vi "1_OnInterrupts.vi"() -> ()   [LabVIEW 2020]
uses:
  <vilib>/Instr/_visa.llb/VISA Configure Serial Port (Instr).vi
  <vilib>/Analysis/NI_AALBase.lvlib
panel:
  in  "stop":bool
  in  "Tab Control":enum32{"Main", "Service"}(tab)
  out "mean":dbl=672.206 format="%.6f"
  out "standard deviation":dbl=7.149110683653894 format="%.6f"
  out "Measurement":dbl(graph)=673.0
  out "error out":errorcluster
  in  "VISA resource name":refnum<visa-resource-name>="COM7"
  out "answer":string="673 \n\r"
  in  "Clear":bool
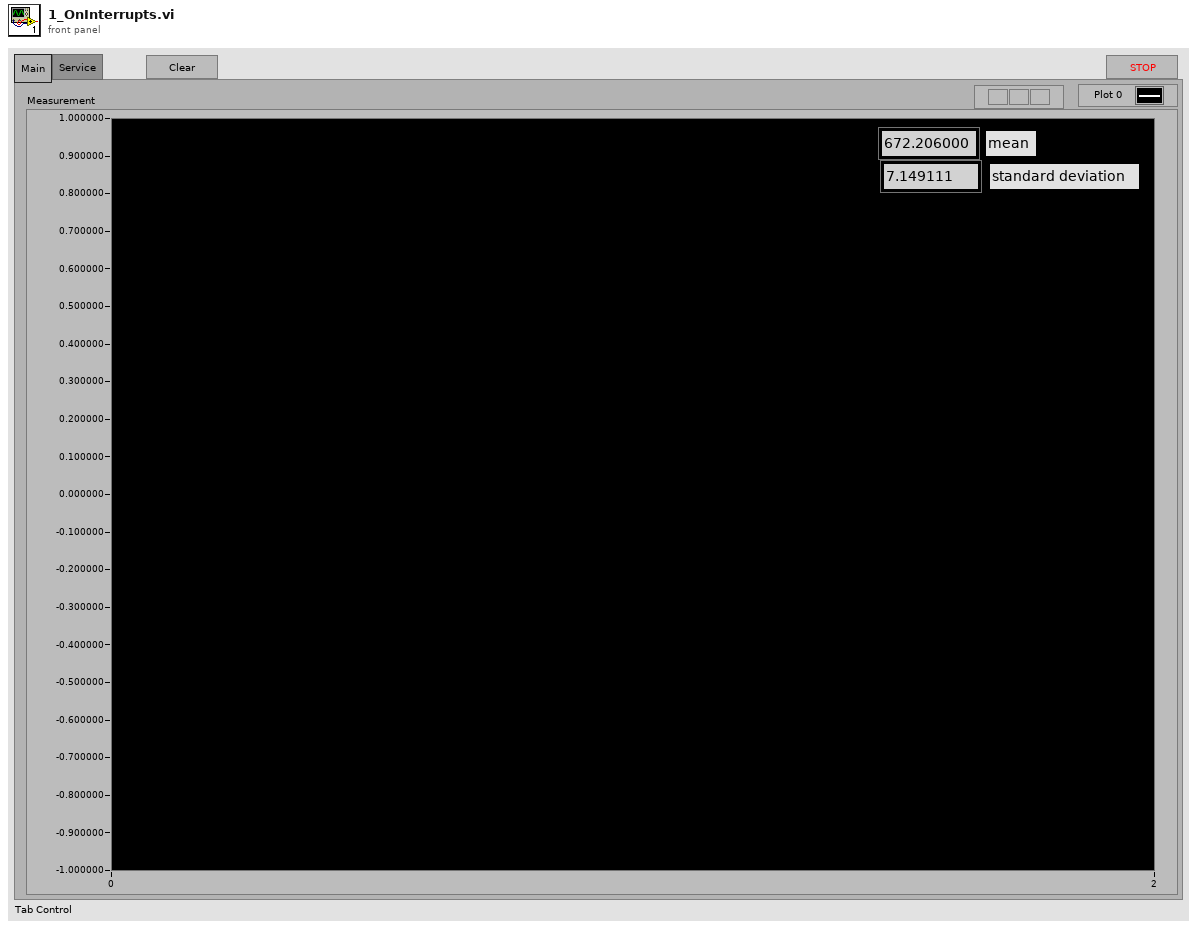
[diagram p1: front panel]
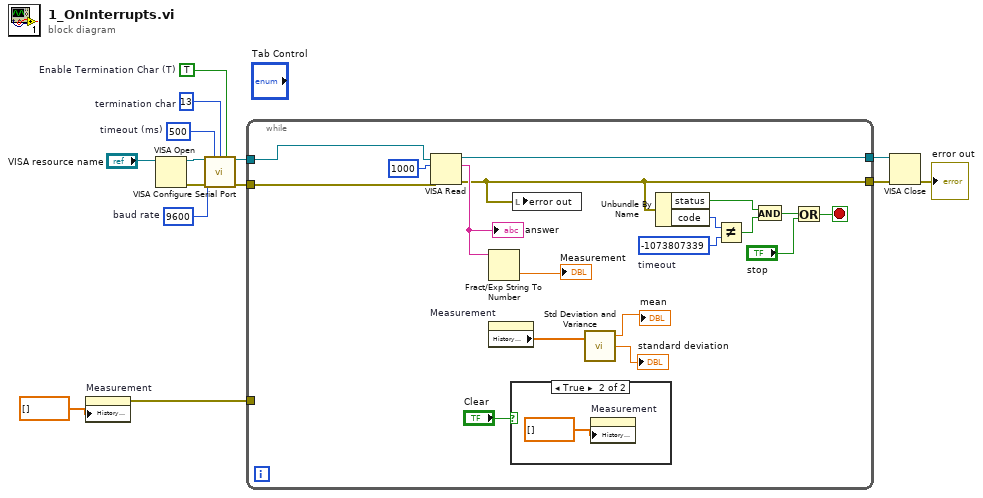
[diagram p0: block diagram]
diagram:
  w3 = u32 9600  # baud rate
  w4 = u32 500  # timeout (ms)
  w10 = TRUE  # Enable Termination Char (T)
  w11 = u8 13  # termination char
  n1 = property on="Measurement" class="WFChart (strict)"("History Data"=dbl[] []) -> (error out=w1:errorcluster)  [unwired: 2 in, 1 out]
  n2 = VISA Open(VISA resource name="VISA resource name") -> (VISA resource name=w13:refnum<visa-resource-name>, error out=w14:errorcluster)  [unwired: 4 in]
  n3 = call-poly "VISA Configure Serial Port"("VISA resource name"=w13, "timeout (10sec)"=w4, "termination char\n(0xA = '\\n' = LF)"=w11, "Enable Termination\nChar (T)"=w10, "baud rate (9600)"=w3, "error in (no error)"=w14) -> ("VISA resource name out"=w7:refnum<visa-resource-name>, "error out"=w6:errorcluster)  [unwired: 8 in]
  n4 = while {
    tunnel: w7 -> [w31]
    tunnel: [w32] -> w9
    tunnel: w6 -> [w15]
    tunnel: [w24] -> w8
    tunnel: w1 -> [_]
    stop <- w18 stop-if-true
    w22 = -1073807339  # timeout
    n5 = VISA Read(VISA resource name=w31, byte count=u32 1000, error in (no error)=w15) -> (VISA resource name out=w32:refnum<visa-resource-name>, read buffer=w29:string, error out=w24:errorcluster)  [unwired: 1 out]
    "answer" <- w29
    n6 = Fract/Exp String To Number(string=w29) -> (number=→"Measurement":dbl)  [unwired: 3 in, 1 out]
    n7 = property on="Measurement" class="WFChart (strict)"() -> ("History Data"=w28:dbl[])  [unwired: 2 in, 2 out]
    n8 = case shown="True" "Clear" {
      frame False {
      }
      frame True {
        n9 = property on="Measurement" class="WFChart (strict)"("History Data"=dbl[] []) -> ()  [unwired: 2 in, 2 out]
      }
    }
    n10 = local write "error out"(w24) -> ()
    n11 = call <vilib>:"Std Deviation and Variance.vi"("X"=w28) -> ("mean"=→"mean":dbl, "standard deviation"=→"standard deviation":dbl)  [unwired: 1 in, 1 out]
    n12 = Unbundle By Name(w24) -> ("status"=w20:bool, "code"=w23:i32)
    n13 = Not Equal?(x=w23, y=w22) -> (x != y?=w21:bool)
    n14 = And(x=w20, y=w21) -> (x .and. y?=w19:bool)
    n15 = Or(x=w19, y="stop") -> (x .or. y?=w18:bool)
  }
  n16 = VISA Close(VISA resource name=w9, error in (no error)=w8) -> (error out=→"error out":errorcluster)
